vi "aal_cascaded moving average (complex input).vi"(1 "Reset":bool, 2 "Stages":i32, 3 "N":i32=1, 4 "x":cdb[](array[numeric])) -> (0 "y":cdb[](array[numeric]))   [LabVIEW 2020, in "NI_AALPro.lvlib"]
uses:
  <vilib>/Analysis/NI_AALPro.lvlib
  <resource>/lvanlys.dll
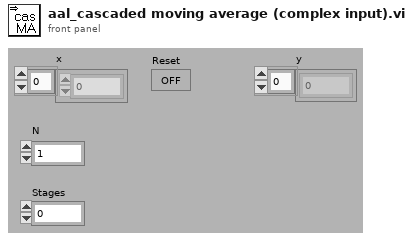
[diagram p1: front panel]
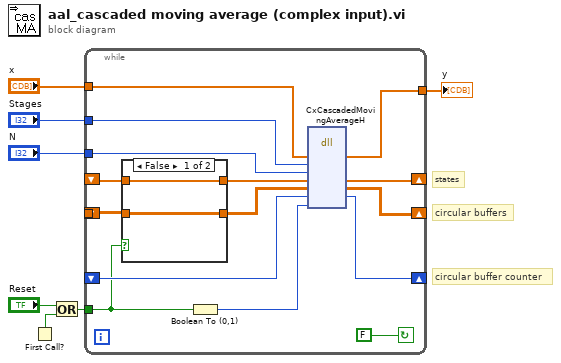
[diagram p0: block diagram]
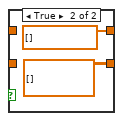
[diagram p2: hidden frame]
diagram:
  # "states"
  # "circular buffers"
  # "circular buffer counter"
  n1 = First Call?() -> (First Call?: T/F=w3:bool)
  n2 = Or(x="Reset", y=w3) -> (x .or. y?=w5:bool)
  n3 = while {
    tunnel: [w8] -> w1
    tunnel: "x" -> [w9]
    tunnel: w5 -> [w13]
    tunnel: [w15] -> _
    tunnel: "Stages" -> [w19]
    tunnel: "N" -> [w20]
    shift-left: _ -> [w15]
    shift-right: [w16] -> _
    shift-left: _ -> [w21]
    shift-right: [w22] -> _
    shift-left: _ -> [w11]
    shift-right: [w10] -> _
    stop <- FALSE continue-if-true
    n4 = case shown="False" w13 {
      tunnel: [w24 cdb[][] [] ("Array Constant")] -> w14
      tunnel: w15 -> [w24 _]
      tunnel: [w23 cdb[] [] ("Array Constant")] -> w12
      tunnel: w11 -> [w23 _]
      frame False {
      }
      frame True {
      }
    }
    n5 = Boolean To (0,1)(Boolean=w13) -> (0, 1=w18:i16)
    n6 = dll-call lib="e:/builds/penguin/labview/branches/2020/dev/dist/resource/lvanlys.*" fn="CxCascadedMovingAverageH"("x"=w9, "stages"=w19, "N"=w20, "Array Constant"=w12, "Array Constant"=w14, "ibuf_cnt"=w21, "Reset"=w18) -> ("x"=w8:cdb[], "Array Constant"=w10:cdb[], "Array Constant"=w16:cdb[][], "ibuf_cnt"=w22:i32)  [unwired: 7 in, 2 out]
  }
  "y" <- w1
